vi "Main - Handle Heirarchy Drag&Drop - Determine Tasks.vi"(8 "error in (no error)":errorcluster, 10 "Drag&Drop Data":T1, 11 "Data in":T2) -> (0 "error out":errorcluster, 3 "Data out":T2, 5 "Copy":bool)   [LabVIEW 2018]
uses:
  TypeDef/Main - Handle Heirarchy Drag&Drop - Data.ctl
  TypeDef/FIlter.ctl
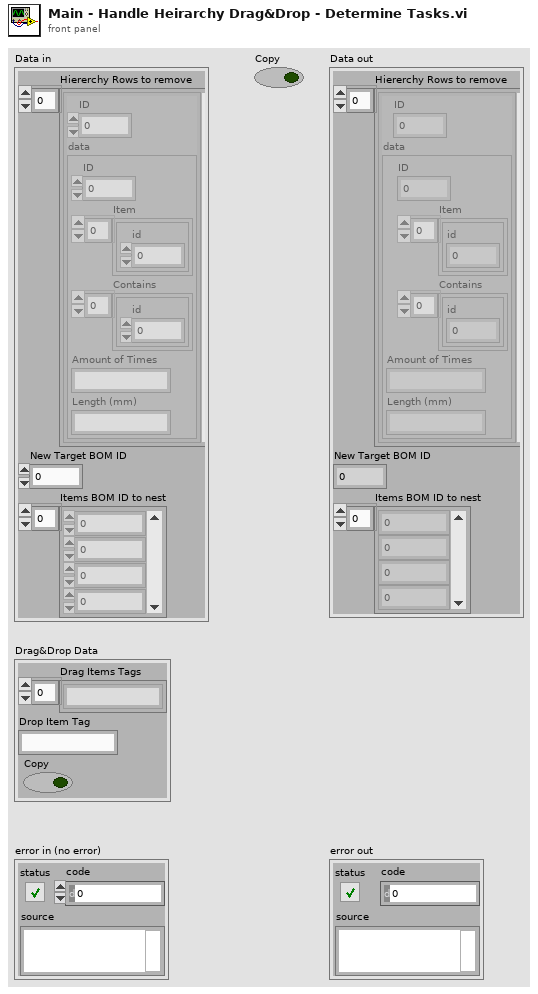
[diagram p1: front panel]
types:
  T1 = cluster{"Drag Items Tags":string[], "Drop Item Tag":string, "Copy":bool}
  T2 = typedef "Main - Handle Heirarchy Drag&Drop - Data.ctl" = cluster{"Hiererchy Rows to remove":cluster{"ID":i32, "data":cluster{"ID":i32, "Item":cluster{"id":i32}[], "Contains":cluster{"id":i32}[], "Amount of Times":string, "Length (mm)":string}}[], "New Target BOM ID":i32, "Items BOM ID to nest":i32[]}
  T3 = typedef "FIlter.ctl" = cluster{"Field Name":string, "Filter Type":string, "Filter Value":string}
  T4 = cluster{"ID":i32, "Item":cluster{"id":i32}[], "Contains":cluster{"id":i32}[], "Amount of Times":string, "Length (mm)":string}
  T5 = cluster{"ID":i32, "data":cluster{"ID":i32, "Item":cluster{"id":i32}[], "Contains":cluster{"id":i32}[], "Amount of Times":string, "Length (mm)":string}}
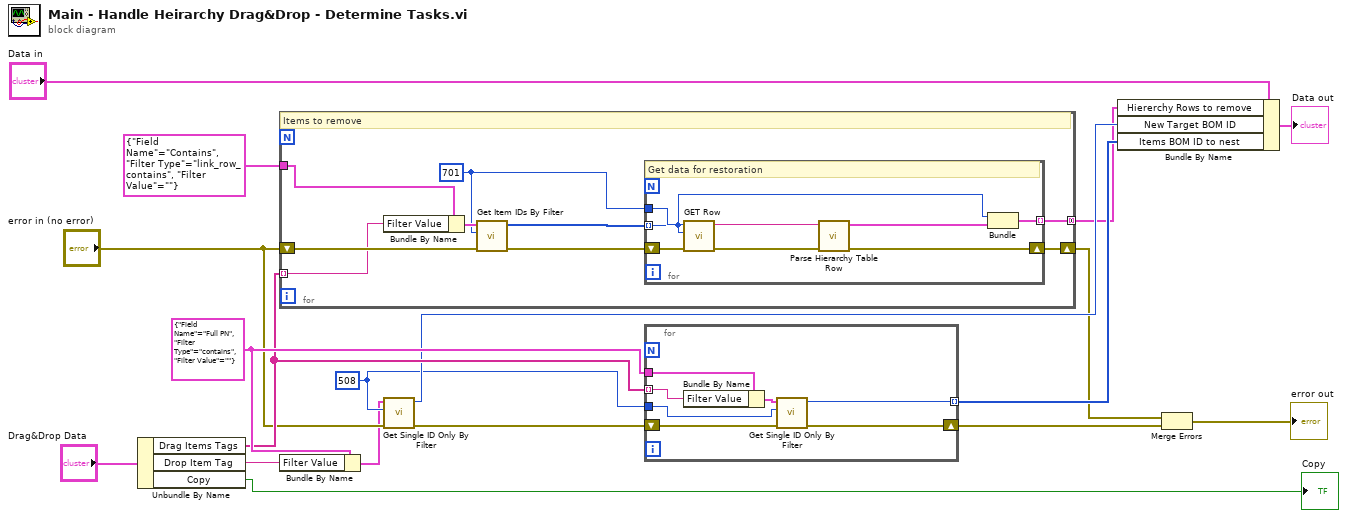
[diagram p0: block diagram]
diagram:
  w9 = u32 508 ("Table ID")
  w18 = T3 {"Field Name"="Full PN", "Filter Type"="contains", "Filter Value"=""} ("Filter")
  n1 = Unbundle By Name("Drag&Drop Data") -> ("Drag Items Tags"=w16:string[], "Drop Item Tag"=w15:string, "Copy"=→"Copy":bool)
  n2 = for {
    tunnel: w16 -> [w26] mode=indexing
    shift-right: [w19] -> w3
    shift-left: "error in (no error)" -> [w27]
    tunnel: [w20] -> w6 mode=concatenating
    tunnel: T3 {"Field Name"="Contains", "Filter Type"="link_row_contains", "Filter Value"=""} ("Filter") -> [w24]
    w23 = u32 701 ("Table ID")
    # "Items to remove"
    n3 = Bundle By Name(cluster=w24, "Filter Value"=w26) -> (w25:T3)
    n4 = call "Get Item IDs By Filter.vi"("error in (no error)"=w27, "Table ID"=w23, "Filter"=w25) -> ("error out"=w22:errorcluster, "Item IDs"=w21:i32[])  [unwired: 7 in]
    n5 = for {
      tunnel: w23 -> [w35]
      tunnel: w21 -> [w31] mode=indexing
      tunnel: [w29] -> w20 mode=indexing
      shift-right: [w28] -> w19
      shift-left: w22 -> [w34]
      # "Get data for restoration"
      n6 = call "GET Row.vi"("Error in"=w34, "Row ID"=w31, "Table ID"=w35) -> ("Error out"=w32:errorcluster, "Rows Array JSON"=w33:string)  [unwired: 7 in]
      n7 = call "Parse Hierarchy Table Row.vi"("Error in"=w32, "Rows Array JSON"=w33) -> ("Error out"=w28:errorcluster, "data"=w30:T4)  [unwired: 8 in]
      n8 = Bundle("ID"=w31, "data"=w30) -> (w29:T5)  [unwired: 1 in]
    }
  }
  n9 = Bundle By Name(cluster=w18, "Filter Value"=w15) -> (w7:T3)
  n10 = call "Get Single ID Only By Filter.vi"("error in (no error)"="error in (no error)", "Table ID"=w9, "Filter"=w7) -> ("error out"=w8:errorcluster, "ID"=w10:i32)  [unwired: 7 in]
  n11 = for {
    tunnel: w16 -> [w41] mode=indexing
    tunnel: w18 -> [w42]
    tunnel: w9 -> [w39]
    shift-right: [w37] -> w13
    shift-left: w8 -> [w38]
    tunnel: [w36] -> w11 mode=indexing
    n12 = Bundle By Name(cluster=w42, "Filter Value"=w41) -> (w40:T3)
    n13 = call "Get Single ID Only By Filter.vi"("error in (no error)"=w38, "Table ID"=w39, "Filter"=w40) -> ("error out"=w37:errorcluster, "ID"=w36:i32)  [unwired: 7 in]
  }
  n14 = Bundle By Name(cluster="Data in", "Hiererchy Rows to remove"=w6, "New Target BOM ID"=w10, "Items BOM ID to nest"=w11) -> (→"Data out":T2)
  n15 = Merge Errors(w3, w13) -> (→"error out":errorcluster)
